vi "LHF.DB.Mongo.Util.ListCollectionV.vi"(6 "$match":string, 7 "type":variant, 8 "error in (no error)":errorcluster, 10 "Collection":string, 11 "LHF.DB.Mongo in":refnum<class "LHF.DB.Mongo.lvclass">) -> (0 "error out":errorcluster, 2 "Documents":variant[](array[variant]), 3 "LHF.DB.Mongo out":refnum<class "LHF.DB.Mongo.lvclass">, 5 "ObjectIDs":string[](array[string]))   [LabVIEW 2013, in "LHF.DB.Mongo.lvclass"]
uses:
  LHF.DB.Mongo.lvclass
  C:/Users/schim/Desktop/Projetos/LabVIEW-MongoDB/src/Driver/MongoDB.Driver.dll
  Driver/MongoDB.Driver.dll
  C:/Users/schim/Desktop/Projetos/LabVIEW-MongoDB/src/Driver/MongoDB.Bson.dll
  Driver/MongoDB.Bson.dll
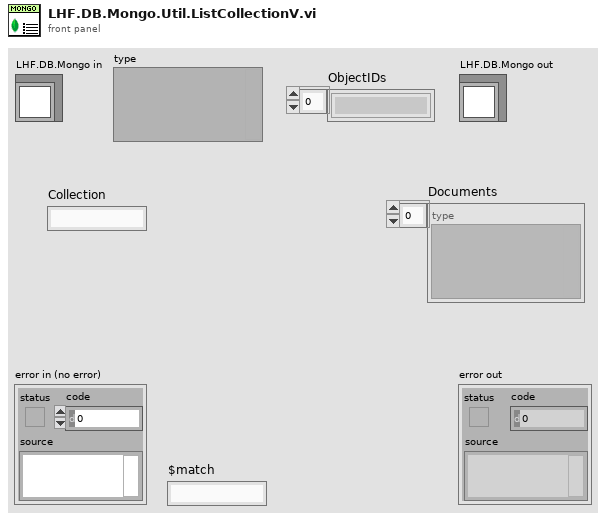
[diagram p1: front panel]
types:
  T1 = typedef "LHF.DB.Mongo.lvclass/LHF.DB.Mongo.Typedef.VariantData.ctl" = cluster{"Type Enum":T2, "Name":string, "Variant":variant}
  T2 = typedef "VariantType.lvlib/Type.ctl" = enum8{"Invalid Type", "Void", "I8", "I16", "I32", "I64", "U8", "U16", "U32", "U64", "Single Float", "Double Float", "Extended Float", "Single Complex", "Double Complex", "Extended Complex", "Enum U8", "Enum U16", "Enum U32", "Enum U64", "Single Float With Unit", "Double Float With Unit", "Extended Float With Unit", "Single Complex with Unit", "Double Complex with Unit", "Extended Complex with Unit", "Boolean", "String", "Path", "Picture", "Tag", "Array", "Cluster", "Variant", "LV Variant", "Waveform", "Timestamp", "Digital Waveform", "Digital Data", "ExpressData", "Refnum", "External Data", "VI", "Poly VI", "LabVIEW Class Instance", "Fixed Point"}
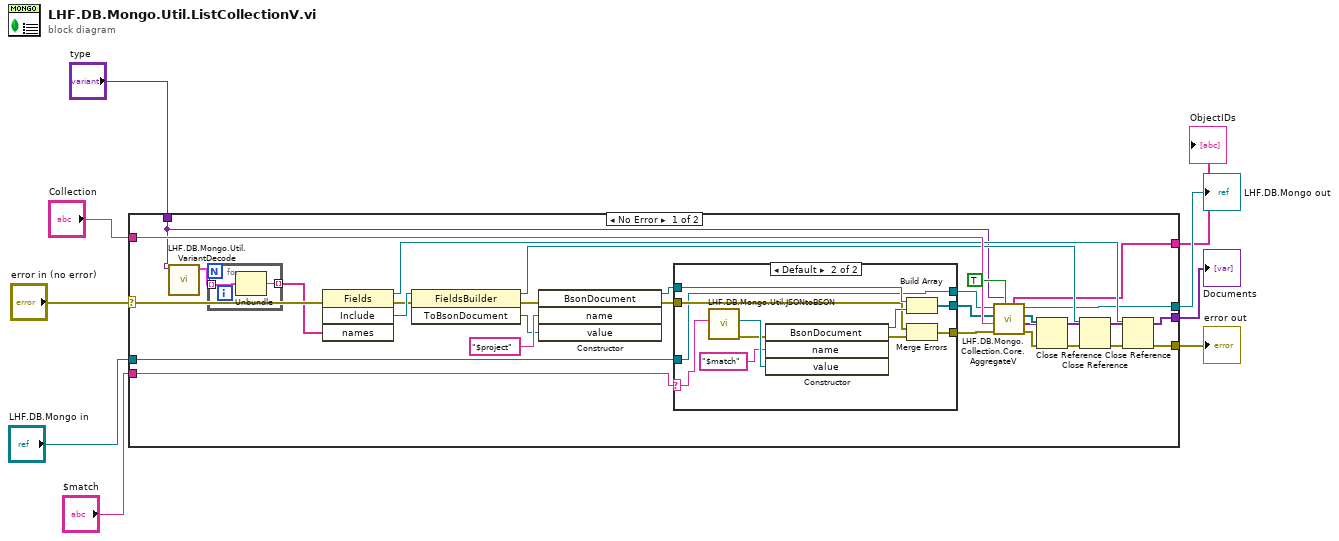
[diagram p0: block diagram]
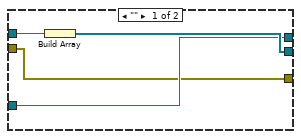
[diagram p2: hidden frame]
diagram:
  n1 = case shown="No Error" "error in (no error)" {
    selector: "error in (no error)" -> [w21 w56]
    tunnel: [w18 w56] -> w8
    tunnel: [w17 w55] -> w6
    tunnel: "LHF.DB.Mongo in" -> [w32 w55]
    tunnel: "Collection" -> [w37 _]
    tunnel: "$match" -> [w15 _]
    tunnel: [w16 _] -> w3
    tunnel: [w13 _] -> w2
    tunnel: "type" -> [w10 _]
    frame No Error {
      n2 = call "LHF.DB.Mongo.Util.VariantDecode.vi"("variant"=w10) -> ("Variant Data"=w12:T1[])  [unwired: 8 in, 2 out]
      n3 = for {
        tunnel: w12 -> [w39] mode=indexing
        tunnel: [w38] -> w11 mode=indexing
        n4 = Unbundle(w39) -> ("Name"=w38:string)  [unwired: 2 out]
      }
      n5 = invoke class="Fields" method="Include"(error in=w21, "names"=w11) -> (reference out=w31:refnum<k24>, error out=w23:errorcluster, "Include"=w35:refnum<k24>)  [unwired: 2 in, 1 out]
      n6 = invoke class="FieldsBuilder" method="ToBsonDocument"(reference=w35, error in=w23) -> (reference out=w30:refnum<k24>, error out=w22:errorcluster, "ToBsonDocument"=w34:refnum<k24>)  [unwired: 1 in]
      n7 = constructor class="BsonDocument"(error in=w22, "name"="$project", "value"=w34) -> (reference out=w33:refnum<k24>, error out=w19:errorcluster)  [unwired: 2 in, 3 out]
      n8 = case shown="Default" w15 {
        selector: w15 -> [_ w45]
        tunnel: w33 -> [w43 w52]
        tunnel: w32 -> [w41 w44]
        tunnel: [w42 w50] -> w29
        tunnel: [w41 w44] -> w28
        tunnel: [w40 w48] -> w20
        tunnel: w19 -> [w40 w46]
        frame "" {
          n9 = Build Array(w43) -> (w42:refnum<k24>[])
        }
        frame Default {
          n10 = call "LHF.DB.Mongo.Util.JSONtoBSON.vi"("JSON data"=w45) -> ("error out"=w49:errorcluster, "BsonValue"=w54:refnum<k24>)  [unwired: 9 in]
          n11 = constructor class="BsonDocument"(error in=w49, "name"="$match", "value"=w54) -> (reference out=w51:refnum<k24>, error out=w47:errorcluster)  [unwired: 2 in, 3 out]
          n12 = Build Array(w52, w51) -> (w50:refnum<k24>[])
          n13 = Merge Errors(w46, w47) -> (w48:errorcluster)
        }
      }
      n14 = call "LHF.DB.Mongo.Collection.Core.AggregateV.vi"("Extract ObjectID"=TRUE ("Extract _id"), "type"=w10, "error in (no error)"=w20, "Collection"=w37, "operations"=w29, "LHF.DB.Mongo in"=w28) -> ("error out"=w26:errorcluster, "Documents"=w16:variant[], "operations out"=w27:refnum<k24>[], "LHF.DB.Mongo out"=w17:refnum<class "LHF.DB.Mongo.lvclass">, "ObjectID"=w13:string[])  [unwired: 1 in]
      n15 = Close Reference(reference=w27, error in (no error)=w26) -> (error out=w25:errorcluster)
      n16 = Close Reference(reference=w30, error in (no error)=w25) -> (error out=w24:errorcluster)
      n17 = Close Reference(reference=w31, error in (no error)=w24) -> (error out=w18:errorcluster)
    }
    frame Error {
    }
  }
  "error out" <- w8
  "LHF.DB.Mongo out" <- w6
  "Documents" <- w3
  "ObjectIDs" <- w2
